vi "connect handshake.vi"(8 "error in":errorcluster, 11 "message":refnum<class "communicator message.lvclass">) -> (0 "error out":errorcluster, 2 "valid?":bool, 3 "queues":T1, 5 "client ID":string)   [LabVIEW 2015, in "Queue server.lvclass"]
uses:
  Queue server.lvclass
  message/communicator message.lvclass
  Queue connection/queue pair.ctl
  message/communicator message.lvclass/communicator message.ctl
  Queue Client/opening handshake data.ctl
  Queue connection/Queue connection.lvclass
  Queue Client/Queue client.lvclass
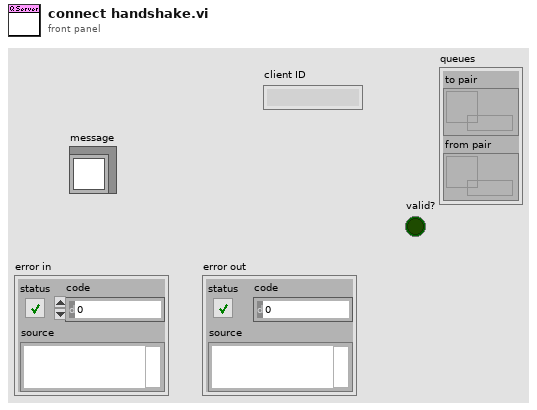
[diagram p1: front panel]
types:
  T1 = typedef "Queue connection.lvclass/queue pair.ctl" = cluster{"to pair":refnum<queue>, "from pair":refnum<queue>}
  T2 = typedef "Queue client.lvclass/opening handshake data.ctl" = cluster{"queue":refnum<queue>, "process ID":string}
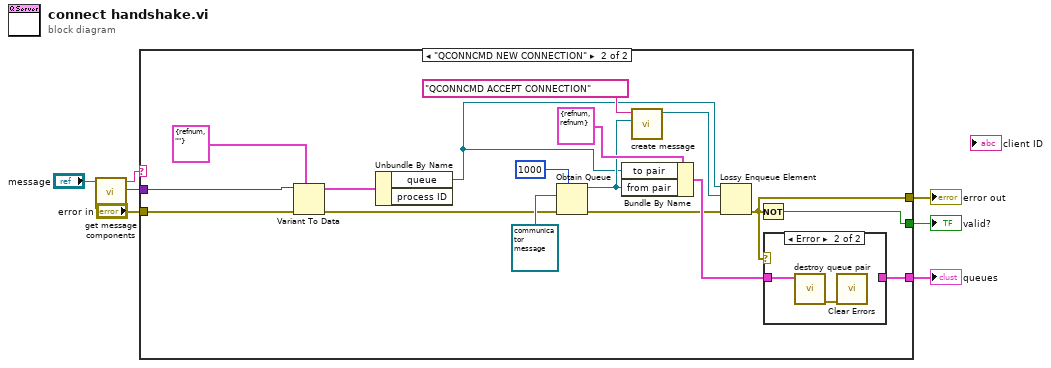
[diagram p0: block diagram]
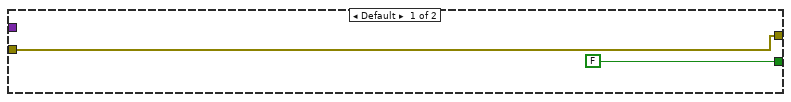
[diagram p2: hidden frame]
diagram:
  n1 = call "get message components.vi"("message"="message") -> ("data"=w2:variant, "ID"=w3:string)  [unwired: 9 in]
  n2 = case shown="\"QCONNCMD NEW CONNECTION\"" w3 {
    tunnel: "error in" -> [w9 w26]
    tunnel: [w9 w16] -> w7
    tunnel: w2 -> [_ w25]
    tunnel: [_ w20] -> w4
    tunnel: [FALSE w17] -> w5
    frame Default {
    }
    frame "QCONNCMD NEW CONNECTION" {
      n3 = Variant To Data(error in=w26, type=T2 {"queue"=refnum, "process ID"=""} ("handshake data"), Variant=w25) -> (data=w19:T2, error out=w23:errorcluster)
      n4 = Unbundle By Name(w19) -> ("queue"=w10:refnum<queue>)  [unwired: 1 out]
      n5 = Obtain Queue(max queue size (-1, unlimited)=1000, element data type=refnum<class "communicator message.lvclass"> refnum ("communicator message.lvclass"), error in (no error)=w23) -> (queue out=w14:refnum<queue>, error out=w18:errorcluster)  [unwired: 2 in, 1 out]
      n6 = Bundle By Name(cluster=T1 {"to pair"=refnum, "from pair"=refnum} ("queues"), "to pair"=w10, "from pair"=w14) -> (w21:T1)
      n7 = call "create message.vi"("data"=w14, "ID"="QCONNCMD ACCEPT CONNECTION") -> ("message"=w12:refnum<class "communicator message.lvclass">)  [unwired: 9 in]
      n8 = Lossy Enqueue Element(queue=w10, element=w12, error in (no error)=w18) -> (error out=w16:errorcluster)  [unwired: 3 out]
      n9 = Not(x=w16) -> (.not. x?=w17:bool)
      n10 = case shown="Error" w16 {
        tunnel: w21 -> [w27 w29]
        tunnel: [w27 _] -> w20
        frame No Error {
        }
        frame Error {
          n11 = call "destroy queue pair.vi"("queue connection"=w29) -> ("error out"=w28:errorcluster)  [unwired: 10 in]
          n12 = call <vilib>:"Clear Errors.vi"("error in (no error)"=w28) -> ()  [unwired: 5 in, 2 out]
        }
      }
    }
  }
  "error out" <- w7
  "valid?" <- w5
  "queues" <- w4
